vi "Initialize Save Header VI.vi"(8 "error in (no error)":errorcluster, 11 "Channel in":refnum<class "Channel.lvclass">) -> (0 "error out":errorcluster, 3 "Channel out":refnum<class "Channel.lvclass">)   [LabVIEW 2018, in "Channel.lvclass"]
uses:
  Channel.lvclass
  Channel.lvclass/Channel.ctl
  Save Image/Save Image.lvclass/Save Image.ctl
  Save Image/Save Image.lvclass
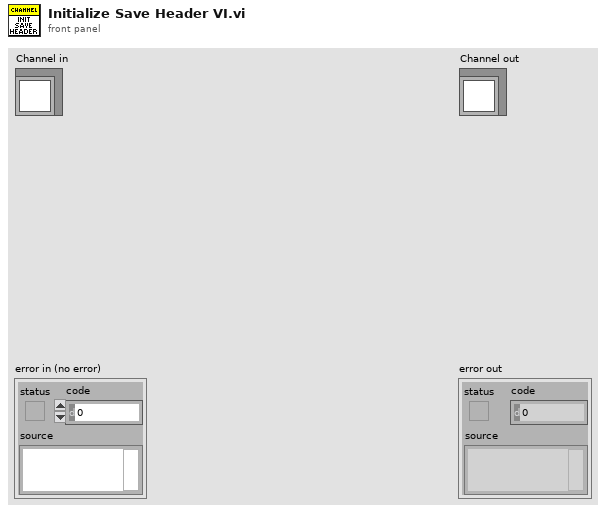
[diagram p1: front panel]
types:
  T1 = cluster{"COMNENT":string, "OBSTYPE":string, "ACSVRSN":string, "CHANNEL":u16, "LAST_IMG_NAME":string, "NIGHTDIR":string}
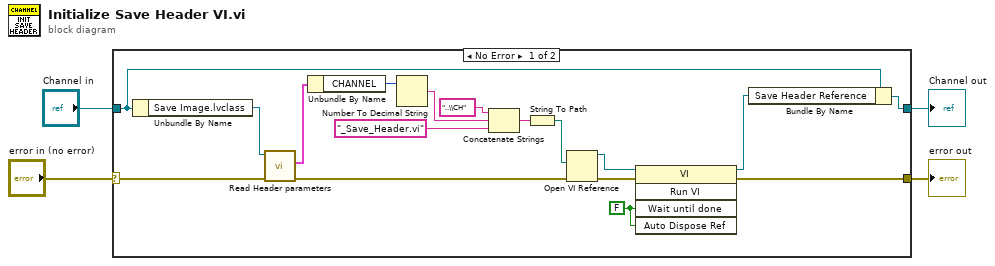
[diagram p0: block diagram]
diagram:
  n1 = case shown="No Error" "error in (no error)" {
    selector: "error in (no error)" -> [w8 w23]
    tunnel: [w16 w23] -> w3
    tunnel: [w11 w22] -> w1
    tunnel: "Channel in" -> [w5 w22]
    frame No Error {
      w20 = FALSE ("Wait Until Done")
      n2 = Unbundle By Name(w5) -> ("Save Image.lvclass"=w10:refnum<class "Save Image.lvclass">)
      n3 = call "Read Header parameters.vi"("error in (no error)"=w8, "Save Image in"=w10) -> ("error out"=w7:errorcluster, "Header parameters"=w9:T1)  [unwired: 7 in, 1 out]
      n4 = Unbundle By Name(w9) -> ("CHANNEL"=w6:u16)
      n5 = Number To Decimal String(number=w6) -> (decimal integer string=w17:string)  [unwired: 1 in]
      n6 = Concatenate Strings("..\\CH" ("name or relative path"), w17, "_Save_Header.vi" ("name or relative path")) -> (w13:string)
      n7 = String To Path(string=w13) -> (path=w14:path)
      n8 = Open VI Reference(vi path=w14, error in (no error)=w7) -> (vi reference=w21:refnum<vi>, error out=w12:errorcluster)  [unwired: 4 in]
      n9 = invoke class="VI" method="Run VI"(reference=w21, error in=w12, "Wait until done"=w20, "Auto Dispose Ref"=w20) -> (reference out=w18:refnum<vi>, error out=w16:errorcluster)  [unwired: 1 in, 3 out]
      n10 = Bundle By Name(cluster=w5, "Save Header Reference"=w18) -> (w11:refnum<class "Channel.lvclass">)
    }
    frame Error {
    }
  }
  "error out" <- w3
  "Channel out" <- w1
